vi "_ExtractArchivedData.vi"(0 "archived_attr_name":string, 1 "from_date":string, 2 "to_date":string, 3 "sampling":string, 4 "db_extractor_dev_name":string) -> (5 "attr values":T1(array[cluster]), 6 "error code":i32, 7 "error stack":string[](array[string]))   [LabVIEW 2014, in "tango.lvlib"]
uses:
  tango.lvlib
  Private VIs/Commands/Insertors/fromDevVarStringArray.vi
  Private VIs/Commands/Extractors/toDevVarLongStringArray.vi
  Private VIs/Commands/Insertors/fromDevString.vi
  tango_binding.so
panel:
  # "This Vi is deprecated and only maintained for backward compatibility. Please use  _TangoExtractArchivedData instead."
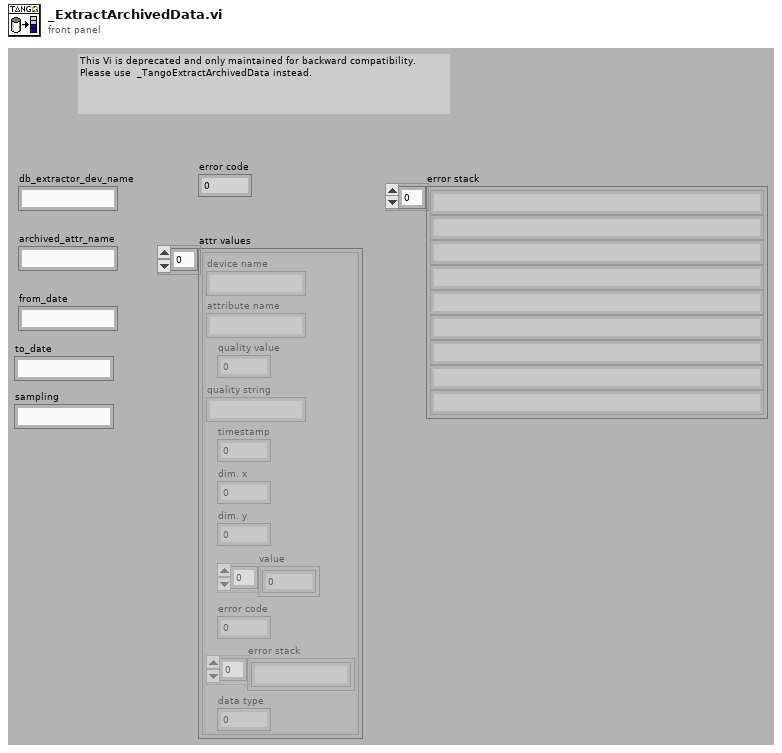
[diagram p1: front panel]
types:
  T1 = cluster{"device name":string, "attribute name":string, "quality value":i16, "quality string":string, "timestamp":dbl, "dim. x":i32, "dim. y":i32, "value":u8[], "error code":i32, "error stack":string[], "data type":u16}[]
  T2 = typedef "tango.lvlib/_AttributeValue_t.ctl" = cluster{"device name":string, "attribute name":string, "quality value":T3, "quality string":string, "timestamp":dbl, "dim. x":i32, "dim. y":i32, "value":u8[], "error code":i32, "error stack":string[], "data type":T4}
  T3 = typedef "tango.lvlib/_AttributeQuality_t.ctl" = enum16{"VALID", "INVALID", "ALARM", "CHANGING", "UNKNOWN_QUALITY"}
  T4 = typedef "tango.lvlib/_AttributeDataType_t.ctl" = enum16{"STATE_SCA", "STATE_SPE", "STATE_IMG", "STRING_SCA", "STRING_SPE", "STRING_IMG", "BOOL_SCA", "BOOL_SPE", "BOOL_IMG", "UCHAR_SCA", "UCHAR_SPE", "UCHAR_IMG", "SHORT_SCA", "SHORT_SPE", "SHORT_IMG", "USHORT_SCA", "USHORT_SPE", "USHORT_IMG", "LONG_SCA", "LONG_SPE", "LONG_IMG", "ULONG_SCA", "ULONG_SPE", "ULONG_IMG", "LONG64_SCA", "LONG64_SPE", "LONG64_IMG", "ULONG64_SCA", "ULONG64_SPE", "ULONG64_IMG", "FLOAT_SCA", "FLOAT_SPE", "FLOAT_IMG", "DOUBLE_SCA", "DOUBLE_SPE", "DOUBLE_IMG", "UNKNOWN_DATA_TYPE"}
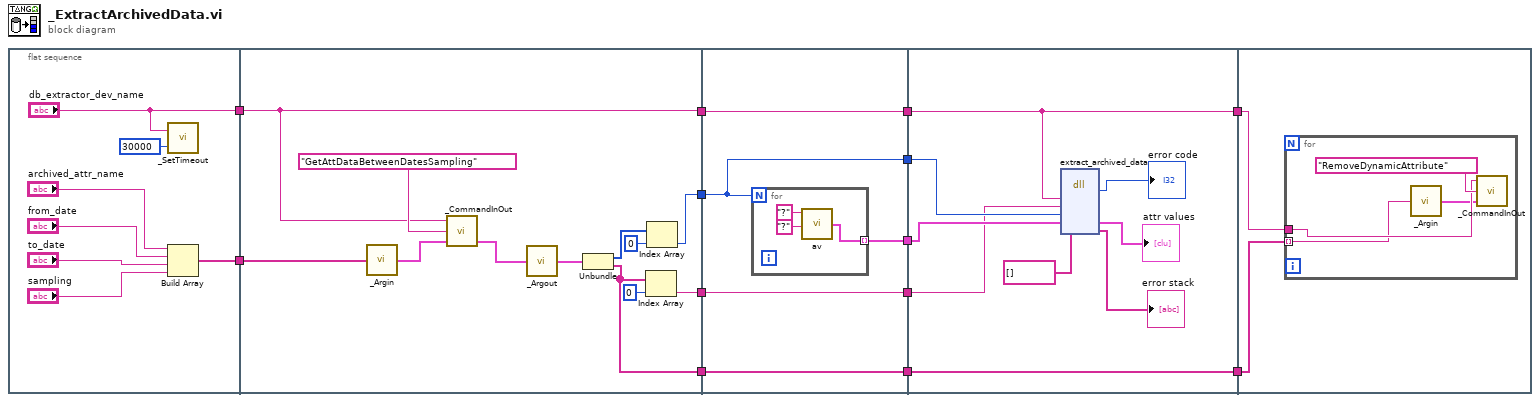
[diagram p0: block diagram]
diagram:
  n1 = flat-sequence {
    tunnel: ["db_extractor_dev_name"] -> w13
    tunnel: [w16] -> w12
    tunnel: w13 -> [w23]
    tunnel: w12 -> [w28]
    tunnel: [w24] -> w11
    tunnel: [w23] -> w8
    tunnel: [w22] -> w6
    tunnel: [w21] -> w1
    tunnel: w11 -> [w34]
    tunnel: [w37] -> w10
    tunnel: [w36] -> w9
    tunnel: w8 -> [w36]
    tunnel: [w35] -> w7
    tunnel: w6 -> [w35]
    tunnel: [w34] -> w5
    tunnel: [w33] -> w2
    tunnel: w1 -> [w33]
    tunnel: w10 -> [w46]
    tunnel: w9 -> [w43]
    tunnel: w7 -> [w44]
    tunnel: w5 -> [w45]
    tunnel: [w43] -> w4
    tunnel: [w41] -> w3
    tunnel: w2 -> [w41]
    tunnel: w4 -> [w51]
    tunnel: w3 -> [w50]
    frame #0 {
      n2 = call "_SetTimeout.vi"("tmo_in_msecs"=u32 30000, "device_name"="db_extractor_dev_name") -> ()  [unwired: 2 out]
      n3 = Build Array("archived_attr_name", "from_date", "to_date", "sampling") -> (w16:string[])
    }
    frame #1 {
      n4 = call-poly "_Argin.vi"("argin"=w28) -> ("ArgIO"=w30:cluster{"num data":u8[], "str data":string[]})
      n5 = call "_CommandInOut.vi"("argin"=w30, "command name"="GetAttDataBetweenDatesSampling", "device name"=w23) -> ("argout"=w31:cluster{"num data":u8[], "str data":string[]})  [unwired: 2 out]
      n6 = call-poly "_Argout.vi"("ArgIO"=w31) -> ("argout"=w32:cluster{"lvalue":i32[], "svalue":string[]})
      n7 = Unbundle(w32) -> ("lvalue"=w27:i32[], "svalue"=w21:string[])
      n8 = Index Array(array=w21, index=0) -> (element=w22:string)
      n9 = Index Array(array=w27, index=0) -> (element=w24:i32)
    }
    frame #2 {
      n10 = for {
        N: w34 -> [_]
        tunnel: [w40] -> w37 mode=indexing
        n11 = call "av.vi"("attribute name"="?", "device name"="?") -> ("attribute value"=w40:T2)  [unwired: 4 in]
      }
    }
    frame #3 {
      n12 = dll-call lib="tango_binding.*" fn="extract_archived_data"("db_extractor_dev_name"=w43, "dynamic_attr_name"=w44, "dynamic_attr_history_len"=w45, "attr_values_inout"=w46, "error_stack"=string[] [] ("error stack")) -> ("return type"=→"error code":i32, "attr_values_inout"=→"attr values":T2[], "error_stack"=→"error stack":string[])  [unwired: 6 in, 2 out]
    }
    frame #4 {
      n13 = for {
        tunnel: w51 -> [w54]
        tunnel: w50 -> [w52] mode=indexing
        n14 = call-poly "_Argin.vi"("argin"=w52) -> ("ArgIO"=w53:cluster{"num data":u8[], "str data":string[]})
        n15 = call "_CommandInOut.vi"("argin"=w53, "command name"="RemoveDynamicAttribute", "device name"=w54) -> ()  [unwired: 3 out]
      }
    }
  }
